vi "test_Series cRIO PWM CAN TC Temp.vi"(8 "Error In":errorcluster) -> (0 "Error Out":errorcluster)   [LabVIEW 2023]
uses:
  Series/Series Base/Series Base.lvclass
  Series/Series Actor/Series Actor/Series Actor.lvclass
  C:/Program Files/National Instruments/LabVIEW 2023/vi.lib/ActorFramework/Actor/Actor.lvclass
  DIO/DO DAQmx Fixed Freq PWM CFG/DO DAQmx Fixed Freq PWM CFG.lvclass
  Sample Tasks/Sample Airtemp PWM Control/Sample Airtemp PWM Control.lvclass
  Devices/NEO480HTA/Real All CFG/Read All CFG.lvclass
  DIO/Virtual DIO/Virt PWM Fixed Freq Generator/Virt PWM Fixed Freq Generator.lvclass
  Thermometer/Thermometer DAQmx Base CFG/Thermometer DAQmx Base CFG.lvclass
  Thermometer/Virtual Thermometers/Virt Temperature Reader/Virt Temperature Reader.lvclass
  Sample Tasks/Sample Watertemp PWM Control/Sample Watertemp PWM Control.lvclass
  Series/Series Base/Series Base.lvclass/Series Base.ctl
  Task/Task Base/Task Base.lvclass/Task Base.ctl
  Series/Series Actor/Series Actor/Series Actor.lvclass/Series Actor.ctl
  <vilib>/ActorFramework/Message Enqueuer/Message Enqueuer.lvclass/Message Enqueuer.ctl
  <vilib>/ActorFramework/Stop Msg/Stop Msg.lvclass/Stop Msg.ctl
  Series/Series Base/Get Task.vi
  <vilib>/ActorFramework/Message Enqueuer/Enqueue.vi
  <vilib>/ActorFramework/Message Enqueuer/Enqueue Critical.vi
  Series/ISeries Actor/ISeries Actor Messages/Start Tasks Msg/Start Tasks Msg.lvclass
  C:/Program Files/National Instruments/LabVIEW 2023/vi.lib/ActorFramework/Message/Message.lvclass
  Series/ISeries Actor/ISeries Actor Messages/Stop Tasks Msg/Stop Tasks Msg.lvclass
  <vilib>/ActorFramework/Stop Msg/Stop Msg.lvclass
  <vilib>/Utility/error.llb/Error Cluster From Error Code.vi
  <vilib>/Utility/LVClass/Get LV Class Name.vi
  <resource>/AFDebug/Generate Trace for Message.vi
  <vilib>/ActorFramework/Message Priority Queue/Priority Enqueue.vi
  <vilib>/ActorFramework/Actor/Actor.lvclass
panel:
  in  "Start Series Button":bool
  in  "Kill Series Actor Button":bool
  out "Temperature Chart Lossy":dbl(graph)
  in  "Temp Setpoint":dbl=23.0 format="%#_g °C"
  in  "stop":bool
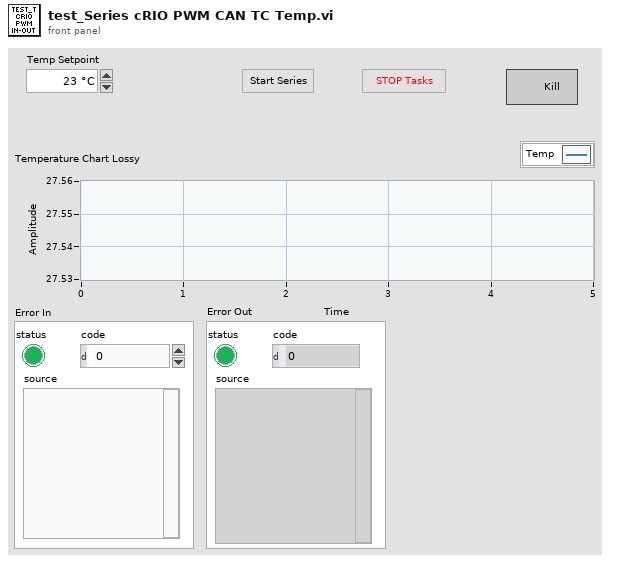
[diagram p1: front panel]
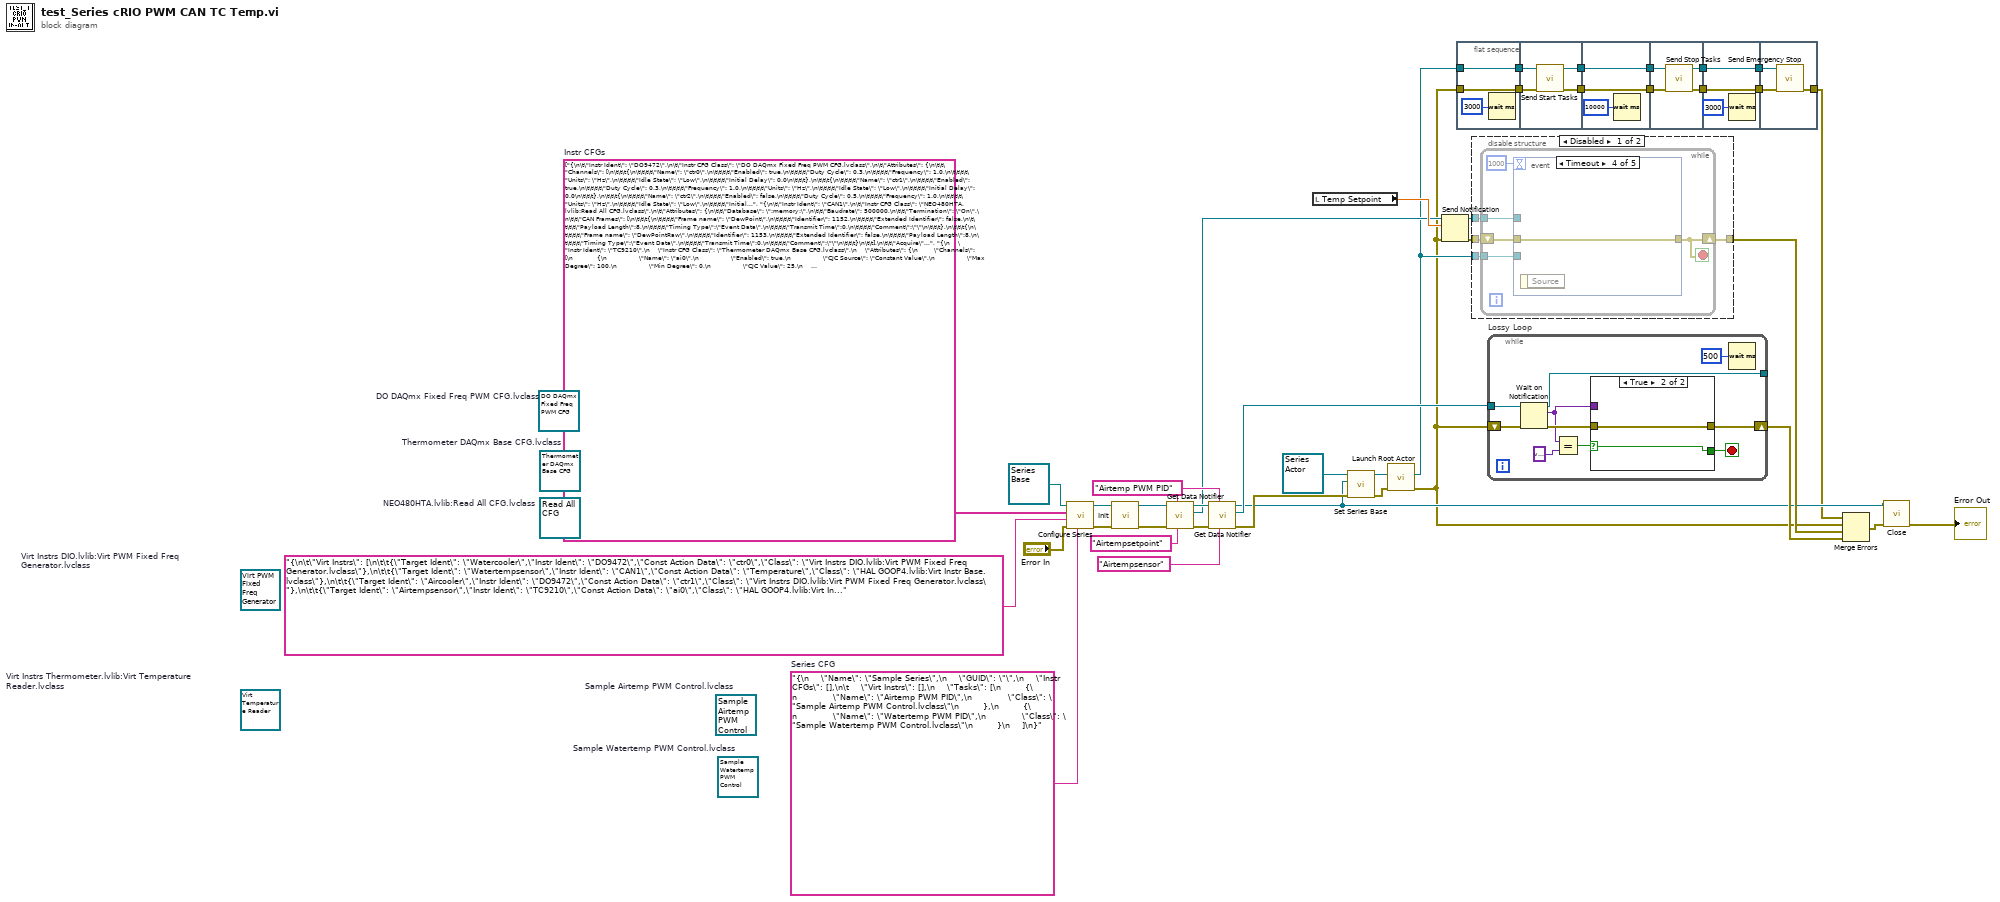
[diagram p0: block diagram]
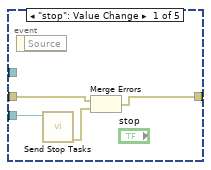
[diagram p2: hidden frame]
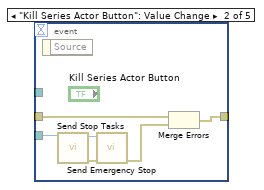
[diagram p3: hidden frame]
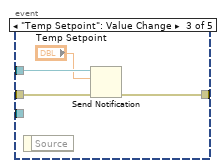
[diagram p4: hidden frame]
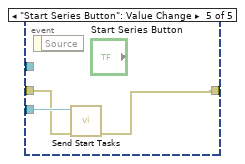
[diagram p5: hidden frame]
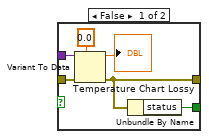
[diagram p7: hidden frame]
diagram:
  (unwired) refnum<class "Sample Watertemp PWM Control.lvclass"> refnum  # Sample Watertemp PWM Control.lvclass
  (unwired) refnum<class "Virt Temperature Reader.lvclass"> refnum  # Virt Instrs Thermometer.lvlib:Virt Temperature Reader.lvclass
  (unwired) refnum<class "Thermometer DAQmx Base CFG.lvclass"> refnum  # Thermometer DAQmx Base CFG.lvclass
  w21 = "Airtemp PWM PID"
  (unwired) refnum<class "Virt PWM Fixed Freq Generator.lvclass"> refnum  # Virt Instrs DIO.lvlib:Virt PWM Fixed Freq Generator.lvclass
  w38 = "{\n    \"Name\": \"Sample Series\",\n    \"GUID\": \"\",\n    \"Instr CFGs\": [],\n\t    \"Virt Instrs\": [],\n    \"Tasks\": [\n        {\n            \"Name\": \"Airtemp PWM PID\",\n            \"Class\": \"Sample Airtemp PWM Control.lvclass\"\n        },\n        {\n            \"Name\": \"Watertemp PWM PID\",\n            \"Class\": \"Sample Watertemp PWM Control.lvclass\"\n        }\n    ]\n}"  # Series CFG
  (unwired) refnum<class "Read All CFG.lvclass"> refnum  # NEO480HTA.lvlib:Read All CFG.lvclass
  (unwired) refnum<class "Sample Airtemp PWM Control.lvclass"> refnum  # Sample Airtemp PWM Control.lvclass
  (unwired) refnum<class "DO DAQmx Fixed Freq PWM CFG.lvclass"> refnum  # DO DAQmx Fixed Freq PWM CFG.lvclass
  w36 = string[] ["{\n\t\"Instr Ident\": \"DO9472\",\n\t\"Instr CFG Class\": \"DO DAQmx Fixed Freq PWM CFG.lvclass\",\n\t\"Attributes\": {\n\t\t\"Channels\": [\n\t\t\t{\n\t\t\t\t\"Name\": \"ctr0\",\n\t\t\t\t\"Enabled\": true,\n\t\t\t\t\"Duty Cycle\": 0.3,\n\t\t\t\t\"Frequency\": 1.0,\n\t\t\t\t\"Units\": \"Hz\",\n\t\t\t\t\"Idle State\": \"Low\",\n\t\t\t\t\"Initial Delay\": 0.0\n\t\t\t},\n\t\t\t{\n\t\t\t\t\"Name\": \"ctr1\",\n\t\t\t\t\"Enabled\": true,\n\t\t\t\t\"Duty Cycle\": 0.3,\n\t\t\t\t\"Frequency\": 1.0,\n\t\t\t\t\"Units\": \"Hz\",\n\t\t\t\t\"Idle State\": \"Low\",\n\t\t\t\t\"Initial Delay\": 0.0\n\t\t\t},\n\t\t\t{\n\t\t\t\t\"Name\": \"ctr2\",\n\t\t\t\t\"Enabled\": false,\n\t\t\t\t\"Duty Cycle\": 0.5,\n\t\t\t\t\"Frequency\": 1.0,\n\t\t\t\t\"Units\": \"Hz\",\n\t\t\t\t\"Idle State\": \"Low\",\n\t\t\t\t\"Initial Delay\": 0.0\n\t\t\t},\n\t\t\t{\n\t\t\t\t\"Name\": \"ctr3\",\n\t\t\t\t\"Enabled\": false,\n\t\t\t\t\"Duty Cycle\": 0.5,\n\t\t\t\t\"Frequency\": 1.0,\n\t\t\t\t\"Units\": \"Hz\",\n\t\t\t\t\"Idle State\": \"Low\",\n\t\t\t\t\"Initial Delay\": 0.0\n\t\t\t}\n\t\t],\n\t\t\"Timing\": {\n\t\t\t\"Samples per Channel\": 1000,\n\t\t\t\"Sample Mode\": \"Continuous Samples\",\n\t\t\t\"Sample Rate\": 0.0,\n\t\t\t\"Sample Clock Source\": \"Implicit\",\n\t\t\t\"Active Edge\": \"Rising\"\n\t\t},\n\t\t\"Trigger\": {\n\t\t\t\"Trigger Type\": \"No Trigger\"\n\t\t}\n\t}\n}", "{\n\t\"Instr Ident\": \"CAN1\",\n\t\"Instr CFG Class\": \"NEO480HTA.lvlib:Read All CFG.lvclass\",\n\t\"Attributes\": {\n\t\t\"Database\": \":memory:\",\n\t\t\"Baudrate\": 500000,\n\t\t\"Termination\": \"On\",\n\t\t\"CAN Frames\": [\n\t\t\t{\n\t\t\t\t\"Frame name\": \"DewPoint\",\n\t\t\t\t\"Identifier\": 1152,\n\t\t\t\t\"Extended Identifier\": false,\n\t\t\t\t\"Payload Length\":8,\n\t\t\t\t\"Timing Type\":\"Event Data\",\n\t\t\t\t\"Transmit Time\":0,\n\t\t\t\t\"Comment\":\"\"\n\t\t\t},\n\t\t\t{\n\t\t\t\t\"Frame name\": \"DewPointRaw\",\n\t\t\t\t\"Identifier\": 1153,\n\t\t\t\t\"Extended Identifier\": false,\n\t\t\t\t\"Payload Length\":8,\n\t\t\t\t\"Timing Type\":\"Event Data\",\n\t\t\t\t\"Transmit Time\":0,\n\t\t\t\t\"Comment\":\"\"\n\t\t\t}\n\t\t],\n\t\t\"Acquire\": {\n\t\t\t\"Type\": \"Read Frame\"\n\t\t}\n\t}\n}", "{\n    \"Instr Ident\": \"TC9210\",\n    \"Instr CFG Class\": \"Thermometer DAQmx Base CFG.lvclass\",\n    \"Attributes\": {\n        \"Channels\": [\n            {\n                \"Name\": \"ai0\",\n                \"Enabled\": true,\n                \"CJC Source\": \"Constant Value\",\n                \"Max Degree\": 100,\n                \"Min Degree\": 0,\n                \"CJC Value\": 25,\n                \"Thermocouple Type\": \"J\",\n                \"Units\": \"Deg C\",\n                \"CJC Channel\": \"\",\n                \"Enable Autozero\": false,\n                \"Autozero Mode\": \"None\"\n            },\n            {\n                \"Name\": \"ai1\",\n                \"Enabled\": false,\n                \"CJC Source\": \"Constant Value\",\n                \"Max Degree\": 100,\n                \"Min Degree\": 0,\n                \"CJC Value\": 25,\n                \"Thermocouple Type\": \"J\",\n                \"Units\": \"Deg C\",\n                \"CJC Channel\": \"\",\n                \"Enable Autozero\": false,\n                \"Autozero Mode\": \"None\"\n            },\n            {\n                \"Name\": \"ai2\",\n                \"Enabled\": false,\n                \"CJC Source\": \"Constant Value\",\n                \"Max Degree\": 100,\n                \"Min Degree\": 0,\n                \"CJC Value\": 25,\n                \"Thermocouple Type\": \"J\",\n                \"Units\": \"Deg C\",\n                \"CJC Channel\": \"\",\n                \"Enable Autozero\": false,\n                \"Autozero Mode\": \"None\"\n            },\n            {\n                \"Name\": \"ai3\",\n                \"Enabled\": false,\n                \"CJC Source\": \"Constant Value\",\n                \"Max Degree\": 100,\n                \"Min Degree\": 0,\n                \"CJC Value\": 25,\n                \"Thermocouple Type\": \"J\",\n                \"Units\": \"Deg C\",\n                \"CJC Channel\": \"\",\n                \"Enable Autozero\": false,\n                \"Autozero Mode\": \"None\"\n            }\n        ],\n        \"Timing\": {\n            \"Samples per Channel\": 1000,\n            \"Sample Mode\": \"Continuous Samples\",\n            \"Sample Rate\": 14,\n            \"Sample Clock Source\": \"OnboardClock\",\n            \"Active Edge\": \"Rising\"\n        },\n        \"Trigger\": {\n            \"Trigger Type\": \"No Trigger\"\n        },\n        \"Acquisition\": {\n            \"Relative To\": \"Current Read Position\",\n            \"Overwrite\": \"Do Not Overwrite Unread Samples\",\n            \"Samples per Fetch\": -1,\n            \"Timeout\": 1\n        }\n    }\n}"]  # Instr CFGs
  n1 = call "Configure Series.vi"("Series CFG"=w38, "error in (no error)"="Error In", "Virt Instrs CFG"="{\n\t\"Virt Instrs\": [\n\t\t{\"Target Ident\": \"Watercooler\",\"Instr Ident\": \"DO9472\",\"Const Action Data\": \"ctr0\",\"Class\": \"Virt Instrs DIO.lvlib:Virt PWM Fixed Freq Generator.lvclass\"},\n\t\t{\"Target Ident\": \"Watertempsensor\",\"Instr Ident\": \"CAN1\",\"Const Action Data\": \"Temperature\",\"Class\": \"HAL GOOP4.lvlib:Virt Instr Base.lvclass\"},\n\t\t{\"Target Ident\": \"Aircooler\",\"Instr Ident\": \"DO9472\",\"Const Action Data\": \"ctr1\",\"Class\": \"Virt Instrs DIO.lvlib:Virt PWM Fixed Freq Generator.lvclass\"},\n\t\t{\"Target Ident\": \"Airtempsensor\",\"Instr Ident\": \"TC9210\",\"Const Action Data\": \"ai0\",\"Class\": \"HAL GOOP4.lvlib:Virt Instr Base.lvclass\"},\n\t]\n}", "Instr CFGs"=w36, "HAL GOOP4:Series Base in"=refnum<class "Series Base.lvclass"> refnum ("HAL GOOP4.lvlib:Study Base.lvclass")) -> ("error out"=w40:errorcluster, "HAL GOOP4:Series Base out"=w41:refnum<class "Series Base.lvclass">)  [unwired: 5 in]
  n2 = call-dynamic "Init.vi"("error in (no error)"=w40, "HAL GOOP4:Series Base in"=w41) -> ("error out"=w34:errorcluster, "HAL GOOP4:Series Base out"=w29:refnum<class "Series Base.lvclass">)  [unwired: 8 in]
  n3 = call "Get Data Notifier.vi"("Data Notifier Name"="Airtempsetpoint" ("Name"), "Task Name"=w21, "error in (no error)"=w34, "Series Base in"=w29) -> ("error out"=w30:errorcluster, "Data Notifier"=w19:refnum<notifier>, "Series Base out"=w23:refnum<class "Series Base.lvclass">)  [unwired: 5 in]
  n4 = call "Get Data Notifier.vi"("Data Notifier Name"="Airtempsensor" ("Target Name"), "Task Name"=w21, "error in (no error)"=w30, "Series Base in"=w23) -> ("error out"=w24:errorcluster, "Data Notifier"=w20:refnum<notifier>, "Series Base out"=w14:refnum<class "Series Base.lvclass">)  [unwired: 5 in]
  n5 = local read "Temp Setpoint"() -> (w31:dbl)
  n6 = call "Set Series Base.vi"("error in (no error)"=w24, "Series Base"=w14, "Series Actor in"=refnum<class "Series Actor.lvclass"> refnum ("Series Actor.lvlib:Series Actor.lvclass")) -> ("error out"=w28:errorcluster, "Series Actor out"=w27:refnum<class "Series Actor.lvclass">)  [unwired: 7 in]
  n7 = call <vilib>:"Launch Root Actor.vi"("error in (no error)"=w28, "Actor"=w27) -> ("error out"=w12:errorcluster, "Actor's Enqueuer"=w13:refnum<class "Message Enqueuer.lvclass">)  [unwired: 8 in]
  n8 = Send Notification(notification=w31, notifier=w19, error in (no error)=w12) -> (notifier out=w18:refnum<notifier>, error out=w32:errorcluster)
  n9 = flat-sequence {
    tunnel: w12 -> [w43]
    tunnel: w13 -> [w44]
    tunnel: [w44] -> w11
    tunnel: [w43] -> w10
    tunnel: w11 -> [w48]
    tunnel: w10 -> [w47]
    tunnel: [w46] -> w9
    tunnel: [w45] -> w8
    tunnel: w9 -> [w50]
    tunnel: w8 -> [w49]
    tunnel: [w50] -> w7
    tunnel: [w49] -> w6
    tunnel: w7 -> [w54]
    tunnel: w6 -> [w55]
    tunnel: [w53] -> w4
    tunnel: [w52] -> w2
    tunnel: [w57] -> w5
    tunnel: w4 -> [w57]
    tunnel: [w56] -> w3
    tunnel: w2 -> [w56]
    tunnel: w5 -> [w60]
    tunnel: w3 -> [w61]
    tunnel: [w59] -> w1
    frame #0 {
      n10 = Wait (ms)(milliseconds to wait=u32 3000) -> ()  [unwired: 1 out]
    }
    frame #1 {
      n11 = call "Send Start Tasks.vi"("error in (no error)"=w47, "Message Enqueuer"=w48) -> ("error out"=w45:errorcluster, "Message Enqueuer out"=w46:refnum<class "Message Enqueuer.lvclass">)  [unwired: 8 in]
    }
    frame #2 {
      n12 = Wait (ms)(milliseconds to wait=u32 10000) -> ()  [unwired: 1 out]
    }
    frame #3 {
      n13 = call "Send Stop Tasks.vi"("error in (no error)"=w55, "Message Enqueuer"=w54) -> ("error out"=w52:errorcluster, "Message Enqueuer out"=w53:refnum<class "Message Enqueuer.lvclass">)  [unwired: 8 in]
    }
    frame #4 {
      n14 = Wait (ms)(milliseconds to wait=u32 3000) -> ()  [unwired: 1 out]
    }
    frame #5 {
      n15 = call <vilib>:"Send Emergency Stop.vi"("error in (no error)"=w61, "Message Enqueuer"=w60) -> ("error out"=w59:errorcluster)  [unwired: 9 in]
    }
  }
  n16 = disable-structure shown="Disabled" {
    disable-tunnel: w32 -> [w65 _]
    disable-tunnel: w18 -> [w64 _]
    disable-tunnel: [w63 _] -> w15
    disable-tunnel: w13 -> [w62 _]
    frame Disabled {
      n17 = while {
        shift-right: [w70] -> w63
        shift-left: w65 -> [w69]
        tunnel: w62 -> [w68]
        tunnel: w64 -> [w67]
        stop <- w70 stop-if-true
        n18 = event shown="[3] Timeout" {
          selector: _ -> [_ _ _ _ _]
          dyn-events: _ -> [_ _ _ _ _]
          timeout: 1000 -> [_ _ _ _ _]
          tunnel: [w71 w78 w82 w85 w86] -> w70
          tunnel: w67 -> [_ _ w84 _ _]
          tunnel: w69 -> [w72 w77 w81 w85 w87]
          tunnel: w68 -> [w74 w80 _ _ w88]
          event "stop": Value Change {
            n19 = event-data() -> ()  [unwired: 1 in, 1 out]
            n20 = call "Send Stop Tasks.vi"("Message Enqueuer"=w74) -> ("error out"=w73:errorcluster)  [unwired: 9 in, 1 out]
            n21 = Merge Errors(w72, w73) -> (w71:errorcluster)
          }
          event "Kill Series Actor Button": Value Change {
            n22 = event-data() -> ()  [unwired: 1 in, 1 out]
            n23 = call "Send Stop Tasks.vi"("Message Enqueuer"=w80) -> ("error out"=w79:errorcluster, "Message Enqueuer out"=w75:refnum<class "Message Enqueuer.lvclass">)  [unwired: 9 in]
            n24 = call <vilib>:"Send Emergency Stop.vi"("error in (no error)"=w79, "Message Enqueuer"=w75) -> ("error out"=w76:errorcluster)  [unwired: 9 in]
            n25 = Merge Errors(w77, w76) -> (w78:errorcluster)
          }
          event "Temp Setpoint": Value Change {
            n26 = event-data() -> ()  [unwired: 1 in, 1 out]
            n27 = Send Notification(notification="Temp Setpoint", notifier=w84, error in (no error)=w81) -> (error out=w82:errorcluster)  [unwired: 1 out]
          }
          event Timeout {
            n28 = event-data() -> ()  [unwired: 1 in, 1 out]
          }
          event "Start Series Button": Value Change {
            n29 = event-data() -> ()  [unwired: 1 in, 1 out]
            n30 = call "Send Start Tasks.vi"("error in (no error)"=w87, "Message Enqueuer"=w88) -> ("error out"=w86:errorcluster)  [unwired: 8 in, 1 out]
          }
        }
      }
    }
    frame Enabled {
    }
  }
  n31 = while "Lossy Loop" {
    tunnel: w20 -> [w94]
    shift-right: [w95] -> w16
    shift-left: w12 -> [w96]
    tunnel: [w93] -> _
    stop <- w92 stop-if-true
    n32 = Wait on Notification(notifier=w94, error in (no error)=w96) -> (notifier out=w93:refnum<notifier>, notification=w90:variant, error out=w98:errorcluster)  [unwired: 2 in, 1 out]
    n33 = Equal?(x=w90, y=variant) -> (x = y?=w89:bool)
    n34 = case shown="True" w89 {
      selector: w89 -> [_ w106]
      tunnel: w98 -> [w104 w105]
      tunnel: [w102 w105] -> w95
      tunnel: [w99 w106] -> w92
      tunnel: w90 -> [w100 _]
      frame False {
        n35 = Variant To Data(error in=w104, type=0.0 ("Waveform"), Variant=w100) -> (data=→"Temperature Chart Lossy":dbl, error out=w102:errorcluster)
        n36 = Unbundle By Name(w102) -> ("status"=w99:bool)
      }
      frame True {
      }
    }
    n37 = Wait (ms)(milliseconds to wait=u32 500) -> ()  [unwired: 1 out]
  }
  n38 = Merge Errors(w1, w12, w15, w16) -> (w17:errorcluster)
  n39 = call-dynamic "Close.vi"("error in (no error)"=w17, "HAL GOOP4:Series Base in"=w14) -> ("error out"=→"Error Out":errorcluster)  [unwired: 8 in, 1 out]
